vi "Acquire Analog Data.vi"() -> ()   [LabVIEW 2023]
uses:
  <vilib>/Platform/TimedLoop/XDataNode/timing_clust.ctl
  <vilib>/Platform/TimedLoop/XDataNode/nitl_modes.ctl
  <vilib>/Platform/TimedLoop/XDataNode/wakeup.ctl
  Type Definitions/Enum - Data.ctl
  Type Definitions/Payload Class.ctl
  Type Definitions/Analog Data.ctl
  <vilib>/Utility/error.llb/Error Cluster From Error Code.vi
  <vilib>/rvi/errors/niLvFpgaAdjustHostInterfaceError.vi
  <vilib>/platform/TimedLoop/XDataNode/XDataNode.xnode
  <vilib>/rvi/interface/nirviReadWriteControl/nirviReadWriteControl.xnode
  <vilib>/rvi/interface/nirviMethod/nirviMethod.xnode
  <vilib>/Platform/TimedLoop/XDataNode/XDNodeRunTimeDep.lvlib
  <vilib>/FPGAPlugInAG/Dynamic/niLvFpga_ReadFifo_Dynamic.vi
  <vilib>/rvi/errors/niLvFpgaMergeErrorWithErrorCode.vi
  <vilib>/rvi/interface/Simulation/niFpgaSimulationCallBeginRW.vi
  NiFpgaLv.dll
  <vilib>/FPGAPlugInAG/Dynamic/niLvFpga_StartFifo_Dynamic.vi
panel:
  out "output array":sgl[][](array[numeric])
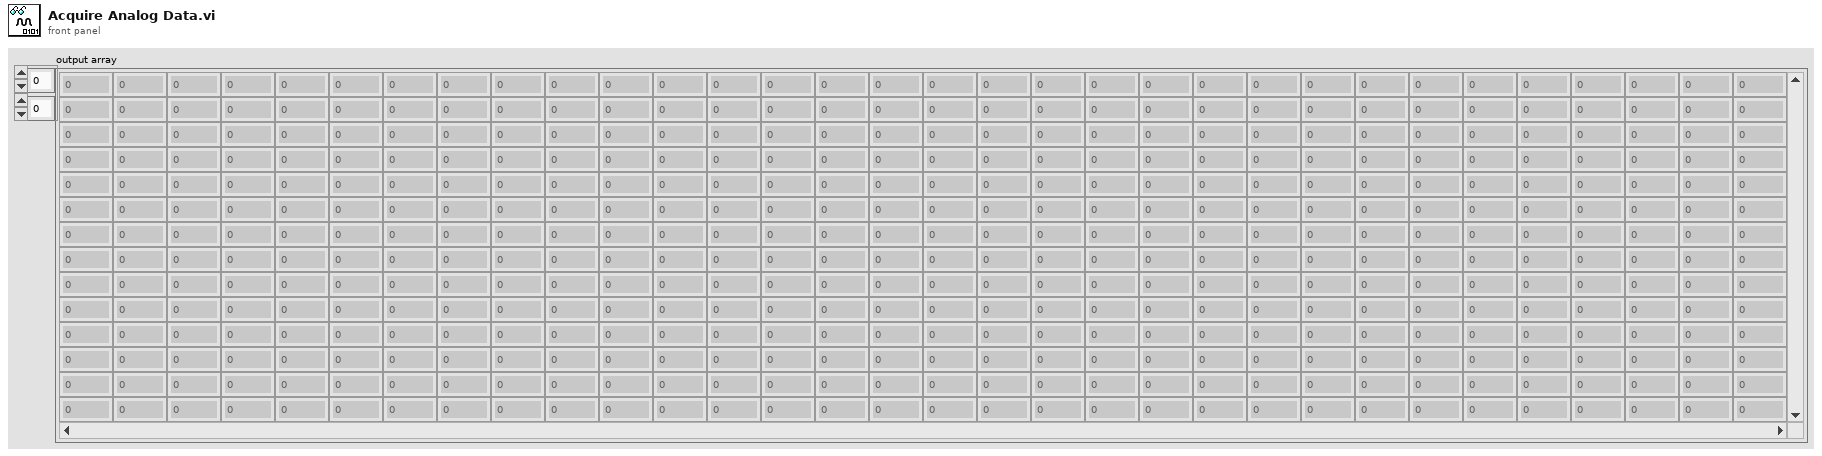
[diagram p1: front panel]
types:
  T1 = typedef "System Resources.ctl" = cluster{"System Session":refnum<k21>, "System Resource":refnum<k20>, "FPGA VI Reference":refnum<k20>}
  T2 = typedef "XDNodeRunTimeDep.lvlib/timing_clust.ctl" = cluster{"Expected End [f-1]":u64, "Actual End [f-1]":u64, "Finished Late? [f-1]":bool, "Expected End [i-1]":u64, "Actual End [i-1]":u64, "Finished Late? [i-1]":bool, "Expected Start [i]":u64, "Actual Start [i]":u64, "Expected Start [f]":u64, "Actual Start [f]":u64, "Source Name":string, "Structure Name":string, "Period":i64, "Deadline":i64, "Offset":i64, "Start":i64, "Priority":i32, "Timeout":i32, "Mode":T3, "Wakeup Reason":T4, "Error":errorcluster, "Source Type":string, "Secondary Source Type":string, "Global End Time":u64, "Global Start Time":u64, "Frame Duration":u64, "Iteration Duration":u64, "Assigned CPU":i32, "I/O Scan Engine Mode":u32}
  T3 = typedef "XDNodeRunTimeDep.lvlib/nitl_modes.ctl" = enum32{"No Change", "Process missed periods, maintain original phase", "Discard missed periods, maintain original phase", "Process missed periods, ignore original phase", "Discard missed periods, ignore original phase"}
  T4 = typedef "XDNodeRunTimeDep.lvlib/wakeup.ctl" = enum32{"Normal", "Aborted", "Asynchronous wakeup", "Timing source error", "Timed loop error", "Timeout"}
  T5 = typedef "Analog Data.ctl" = cluster{"Analog Data":sgl[][]}
  T6 = typedef "Payload Class.ctl" = enum16{"System State", "Parameters", "Metadata", "Software Monitor", "Data", "Commands"}
  T7 = typedef "Enum - Data.ctl" = enum16{"Analog Input Data", "Notification Data", "Analog Output Data", "Digital Output Data", "Command Ack", "Digital Input Data", "GPS Solution Data"}
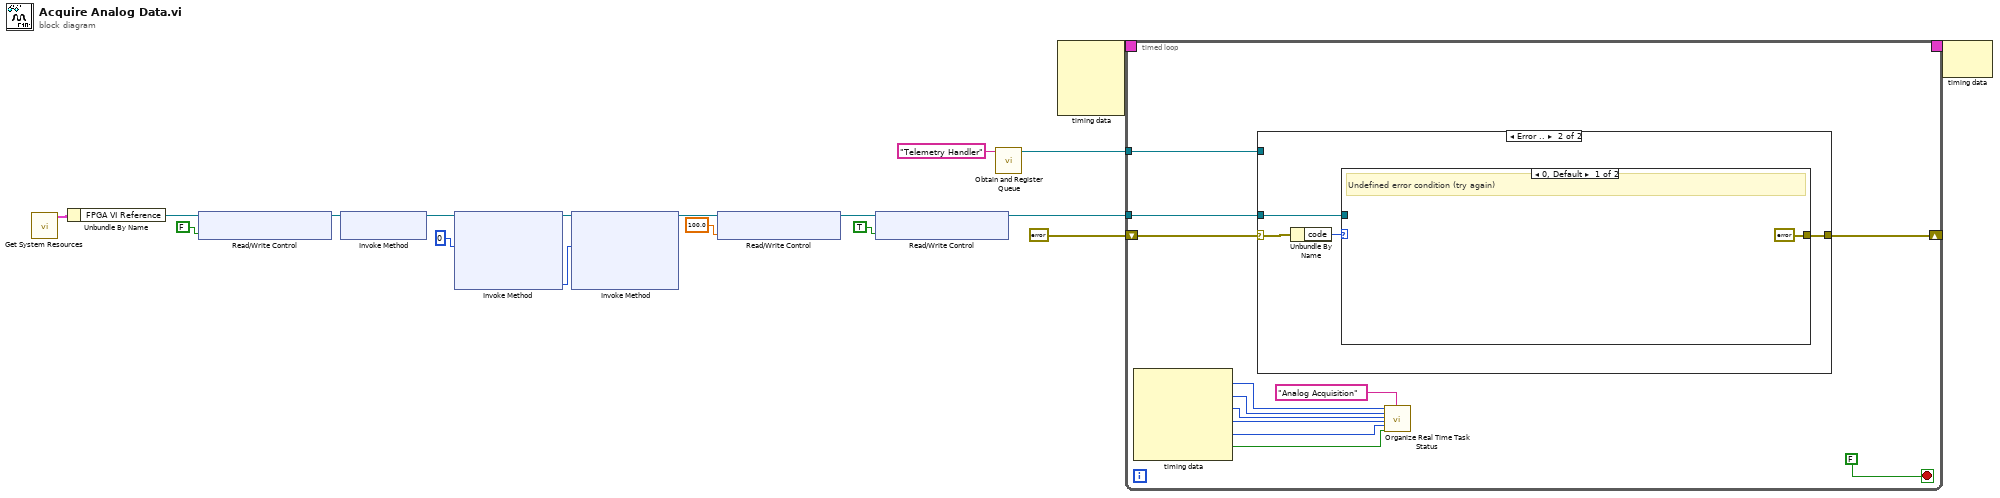
[diagram p0: block diagram]
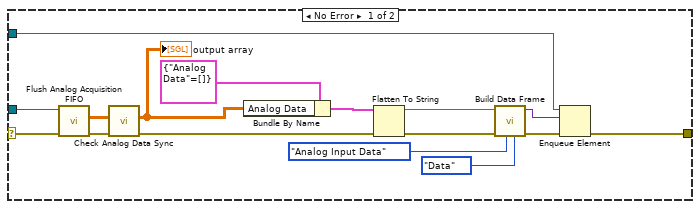
[diagram p2: hidden frame]
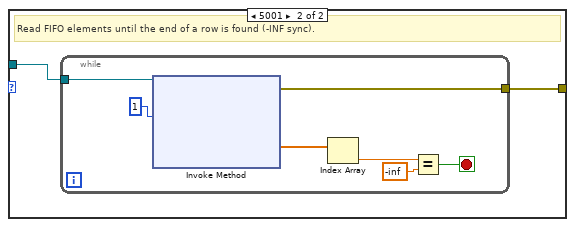
[diagram p3: hidden frame]
diagram:
  n1 = call "Get System Resources.vi"() -> ("System Resources"=w3:T1)  [unwired: 10 in, 1 out]
  n2 = Unbundle By Name(w3) -> ("FPGA VI Reference"=w6:refnum<k20>)
  n3 = xnode "Read/Write Control"("FPGA VI Reference In"=w6, "Enable Analog Acquisition"=FALSE ("Enable Acquisition")) -> ("FPGA VI Reference Out"=w8:refnum<k20>)  [unwired: 1 in, 1 out]
  n4 = xnode "Invoke Method"("FPGA VI Reference In"=w8) -> ("FPGA VI Reference Out"=w9:refnum<k20>)  [unwired: 1 in, 1 out]
  n5 = xnode "Invoke Method"("FPGA VI Reference In"=w9, "Number of Elements"=u32 0) -> ("FPGA VI Reference Out"=w12:refnum<k20>, "Elements Remaining"=w11:u32)  [unwired: 2 in, 2 out]
  n6 = xnode "Invoke Method"("FPGA VI Reference In"=w12, "Number of Elements"=w11) -> ("FPGA VI Reference Out"=w13:refnum<k20>)  [unwired: 2 in, 3 out]
  n7 = xnode "Read/Write Control"("FPGA VI Reference In"=w13, "Analog Acquisition Rate"=sgl 100.0 ("Acquisition Rate (10,000 Hz)")) -> ("FPGA VI Reference Out"=w14:refnum<k20>)  [unwired: 1 in, 1 out]
  n8 = xnode "Read/Write Control"("FPGA VI Reference In"=w14, "Enable Analog Acquisition"=TRUE ("Enable Acquisition")) -> ("FPGA VI Reference Out"=w1:refnum<k20>)  [unwired: 1 in, 1 out]
  n9 = call "Obtain and Register Queue.vi"("Queue Name (unnamed)"="Telemetry Handler" ("name (unnamed)")) -> ("Queue Reference"=w4:refnum<queue>)  [unwired: 9 in, 1 out]
  n10 = node-c288() -> (w18:T2)  [unwired: 4 in]
  n11 = timed-loop {
    timing: w18 -> [_]
    timing-out: [_] -> w17
    tunnel: w4 -> [w22]
    tunnel: w1 -> [w23]
    shift-right: [w20] -> _
    shift-left: errorcluster {"status"=FALSE, "code"=0, "source"=""} ("error out") -> [w19]
    stop <- FALSE stop-if-true
    n12 = node-c288() -> (w28:i32, w27:i32, w26:i64, w21:i64, w25:i64, w24:bool)  [unwired: 1 in]
    n13 = case shown="Error .." w19 {
      selector: w19 -> [w31 w48]
      tunnel: w23 -> [w46 w50]
      tunnel: w22 -> [w45 _]
      tunnel: [w36 w49] -> w20
      frame No Error {
        n14 = call "Flush Analog Acquisition FIFO.vi"("error in"=w31, "FPGA VI Reference"=w46) -> ("error out"=w39:errorcluster, "Analog Data"=w40:sgl[][])  [unwired: 7 in, 1 out]
        n15 = call "Check Analog Data Sync.vi"("error in (no error)"=w39, "Analog Data"=w40) -> ("error out"=w33:errorcluster, "Analog Data Out"=w32:sgl[][])  [unwired: 8 in]
        "output array" <- w32
        n16 = Bundle By Name(cluster=T5 {"Analog Data"=[]} ("Analog Data"), "Analog Data"=w32) -> (w34:T5)
        n17 = Flatten To String(anything=w34, error in (no error)=w33) -> (data string=w44:string, error out=w38:errorcluster)  [unwired: 2 in, 1 out]
        n18 = call "Build Data Frame.vi"("Payload Class (Data)"=Payload_Class."Data", "Payload ID (0)"=Enum_-_Data."Analog Input Data" ("Data"), "error in (no error)"=w38, "Payload (Empty String)"=w44) -> ("error out"=w37:errorcluster, "Frame"=w41:variant)  [unwired: 6 in]
        n19 = Enqueue Element(queue=w45, element=w41, error in (no error)=w37) -> (error out=w36:errorcluster)  [unwired: 1 in, 2 out]
      }
      frame Error {
        n20 = Unbundle By Name(w48) -> ("code"=w47:i32)
        n21 = case shown="0, Default" w47 {
          tunnel: w50 -> [_ w53]
          tunnel: [errorcluster {"status"=FALSE, "code"=0, "source"=""} ("error out") w52] -> w49
          frame 0, Default {
            # "Undefined error condition (try again)"
          }
          frame 5001 {
            # "Read FIFO elements until the end of a row is found (-INF sync)."
            n22 = while {
              tunnel: w53 -> [w60]
              tunnel: [w54] -> w52
              stop <- w55 stop-if-true
              n23 = xnode "Invoke Method"("FPGA VI Reference In"=w60, "Number of Elements"=u32 1) -> ("error out"=w54:errorcluster, "Data"=w58:sgl[])  [unwired: 2 in, 2 out]
              n24 = Index Array(array=w58) -> (element=w57:sgl)  [unwired: 1 in]
              n25 = Equal?(x=w57, y=sgl -inf) -> (x = y?=w55:bool)
            }
          }
        }
      }
    }
    n26 = call "Organize Real Time Task Status.vi"("Priority"=w28, "Processor"=w27, "Offset"=w26, "Iteration Duration"=w21, "Period"=w25, "Finished Late? [i-1]"=w24, "Task Name"="Analog Acquisition") -> ()  [unwired: 12 in, 1 out]
  }
  n27 = node-c288(w17) -> ()  [unwired: 1 out]
